vi "Countdown_Function.vi"(8 "error in (no error)":errorcluster) -> (0 "error out":errorcluster, 2 "Stop?":bool)   [LabVIEW 2018]
doc: "Thsi VI allows user to prepare before the test commences. \n\nInput:\nError In.\n\nOutputs:\nStop?;\nError Out."
panel:
  in  "Stop":bool
  out "Please get ready\nThe test is about to begin":u32(knob)=5 scale=0.0..5.0
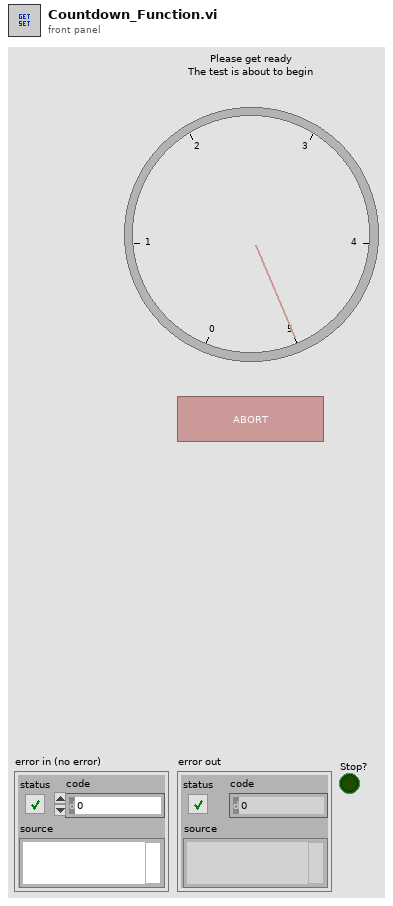
[diagram p1: front panel]
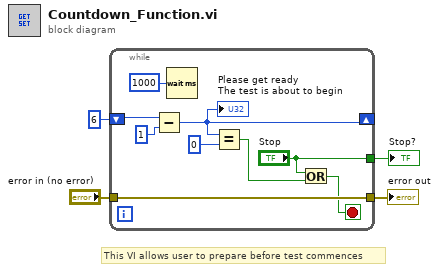
[diagram p0: block diagram]
diagram:
  # "This VI allows user to prepare before test commences"
  n1 = while {
    shift-right: [w9] -> _
    shift-left: u32 6 -> [w10]
    tunnel: "error in (no error)" -> [w8]
    tunnel: [w8] -> w2
    tunnel: ["Stop"] -> w1
    stop <- w7 stop-if-true
    n2 = Subtract(x=w10, y=u32 1) -> (x-y=w9:u32)
    "Please get ready\nThe test is about to begin" <- w9
    n3 = Wait (ms)(milliseconds to wait=u32 1000) -> ()  [unwired: 1 out]
    n4 = Equal?(x=w9, y=u32 0) -> (x = y?=w6:bool)
    n5 = Or(x="Stop", y=w6) -> (x .or. y?=w7:bool)
  }
  "error out" <- w2
  "Stop?" <- w1
